vi "TimeStampAsISO8601Value.vi"(8 "error in":errorcluster, 11 "time stamp":timestamp) -> (0 "error out":errorcluster, 3 "scalar string":string)   [LabVIEW 2014]
doc: "Format a LV timestamp as an XML-RPC formatted ISO8601 time"
panel:
  in  "time format string (%c)":string="%Y-%m-%dT%H:%M:%SZ"
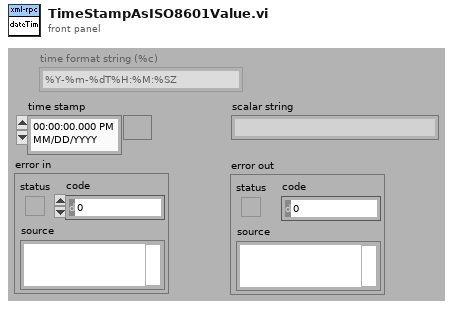
[diagram p1: front panel]
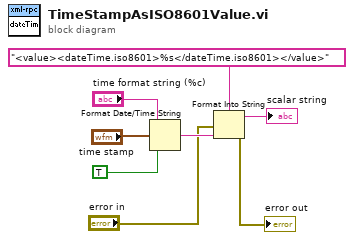
[diagram p0: block diagram]
diagram:
  n1 = Format Date/Time String(time format string (%c)="time format string (%c)", seconds (now)="time stamp", UTC format=TRUE) -> (date/time string=w5:string)
  n2 = Format Into String(format string="<value><dateTime.iso8601>%s</dateTime.iso8601></value>", error in="error in", w5) -> (resulting string=→"scalar string":string, error out=→"error out":errorcluster)  [unwired: 1 in]
